vi "PQescapeStringConn.vi"(0 "conn":u32, 5 "to":string, 7 "from":string, 9 "error":i32, 11 "length":u32, 12 "error in (no error)":errorcluster) -> (4 "conn_out":u32, 6 "size_t":u32, 8 "pq_error_out":i32, 15 "error out":errorcluster)   [LabVIEW 2019, in "libpqlv.lvlib"]
uses:
  libpqlv.lvlib
  libpq.dll
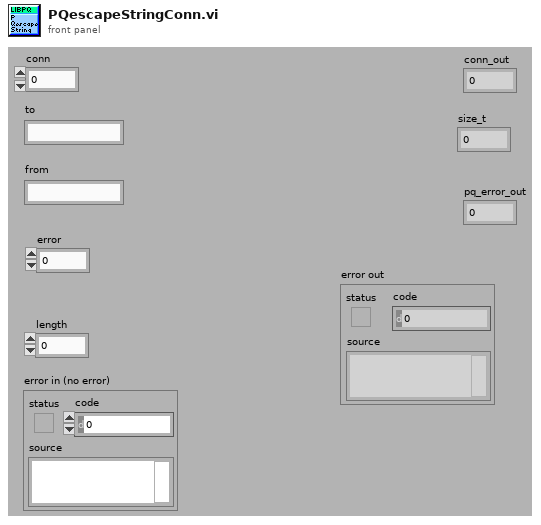
[diagram p1: front panel]
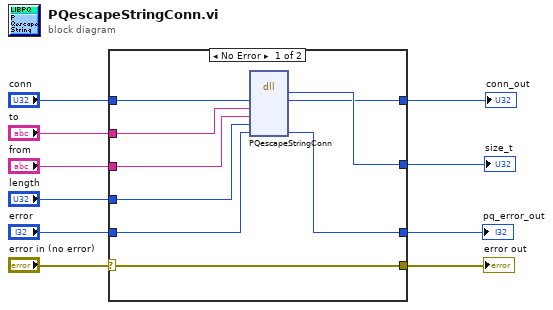
[diagram p0: block diagram]
diagram:
  n1 = case shown="No Error" "error in (no error)" {
    selector: "error in (no error)" -> [w19 w22]
    tunnel: [w19 w22] -> w9
    tunnel: [w18 _] -> w8
    tunnel: [w17 w21] -> w3
    tunnel: "to" -> [w16 _]
    tunnel: "from" -> [w15 _]
    tunnel: "length" -> [w14 _]
    tunnel: "error" -> [w13 w20]
    tunnel: "conn" -> [w12 w21]
    tunnel: [w11 w20] -> w1
    frame No Error {
      n2 = dll-call lib="libpq.*" fn="PQescapeStringConn"("conn"=w12, "to"=w16, "from"=w15, "length"=w14, "error"=w13) -> ("size_t"=w18:u32, "conn"=w17:u32, "error"=w11:i32)  [unwired: 6 in, 2 out]
    }
    frame Error {
    }
  }
  "size_t" <- w8
  "error out" <- w9
  "conn_out" <- w3
  "pq_error_out" <- w1
